vi "Online_Statistic_Initialize.vi"(8 "error in (no error)":errorcluster, 11 "Online_Statistic in":refnum<class "Online_Statistic.lvclass">) -> (0 "error out":errorcluster, 3 "Online_Statistic out":refnum<class "Online_Statistic.lvclass">)   [LabVIEW 2021, in "Online_Statistic.lvclass"]
uses:
  Online_Statistic.lvclass
  Online_Statistic.lvclass/Online_Statistic.ctl
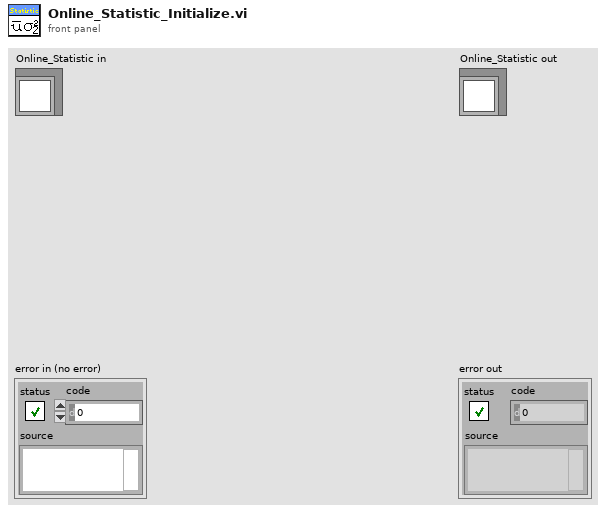
[diagram p1: front panel]
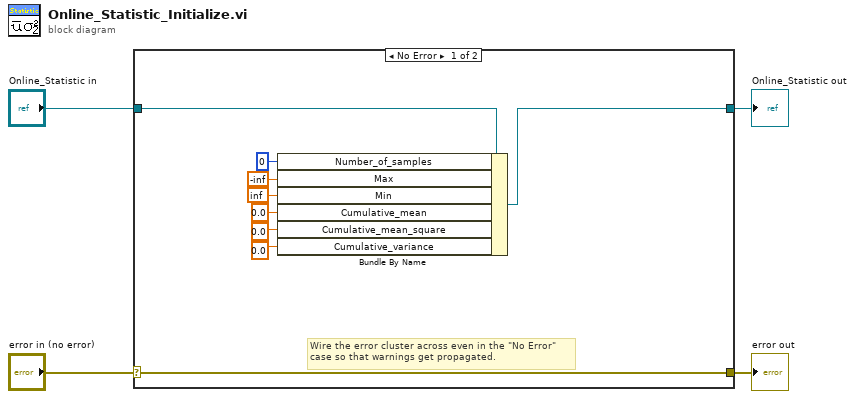
[diagram p0: block diagram]
diagram:
  n1 = case shown="No Error" "error in (no error)" {
    selector: "error in (no error)" -> [w13 w15]
    tunnel: [w13 w15] -> w3
    tunnel: [w5 w14] -> w1
    tunnel: "Online_Statistic in" -> [w12 w14]
    frame No Error {
      # "Wire the error cluster across even in the \"No Error\"\ncase so that warnings get propagated."
      n2 = Bundle By Name(cluster=w12, "Number_of_samples"=0 ("stats_private.Number_of_samples"), "Max"=-inf, "Min"=inf, "Cumulative_mean"=0.0 ("stats_private.Cumulative_mean"), "Cumulative_mean_square"=0.0 ("stats_private.Cumulative_mean"), "Cumulative_variance"=0.0 ("stats_private.Cumulative_mean")) -> (w5:refnum<class "Online_Statistic.lvclass">)
    }
    frame Error {
    }
  }
  "error out" <- w3
  "Online_Statistic out" <- w1
